vi "sort module schedule.vi"(11 "priority array":T1(array[cluster])) -> (3 "sorted module indices":i32[](array[numeric]))   [LabVIEW 2013, in "Standard Engine Runtime.lvclass"]
uses:
  Standard Engine Runtime.lvclass
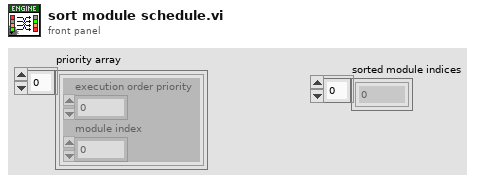
[diagram p1: front panel]
types:
  T1 = cluster{"execution order priority":i32, "module index":i32}[]
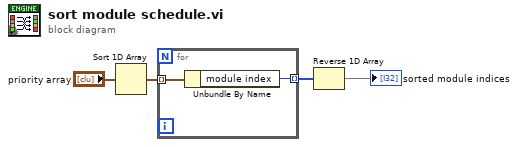
[diagram p0: block diagram]
diagram:
  n1 = Sort 1D Array(array="priority array") -> (sorted array=w3:T1)
  n2 = for {
    tunnel: w3 -> [w6] mode=indexing
    tunnel: [w5] -> w2 mode=indexing
    n3 = Unbundle By Name(w6) -> ("module index"=w5:i32)
  }
  n4 = Reverse 1D Array(array=w2) -> (reversed array=→"sorted module indices":i32[])
